vi "Pop Timings Header.vi"(8 "error in (no error)":errorcluster, 11 "Header in":refnum<class "Simulated_Header.lvclass">) -> (0 "error out":errorcluster, 2 "timings header":string, 3 "Header out":refnum<class "Simulated_Header.lvclass">)   [LabVIEW 2018, in "Simulated_Header.lvclass"]
uses:
  Simulated_Header.lvclass
  Simulated_Header.lvclass/Simulated_Header.ctl
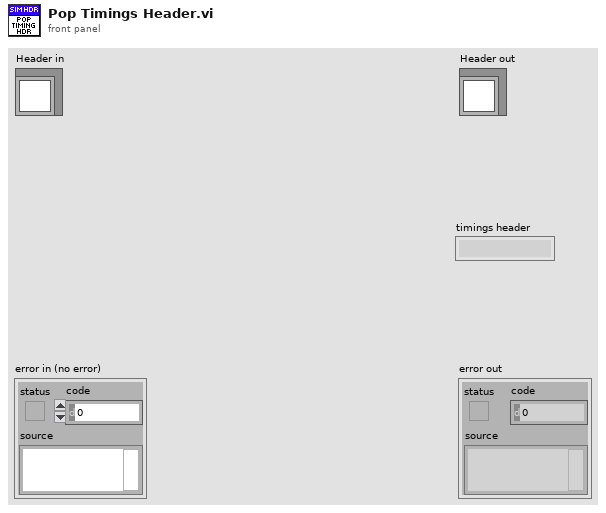
[diagram p1: front panel]
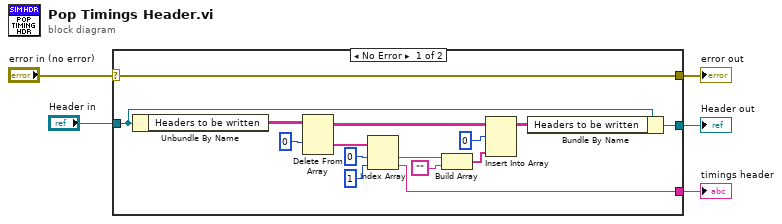
[diagram p0: block diagram]
diagram:
  n1 = case shown="No Error" "error in (no error)" {
    selector: "error in (no error)" -> [w10 w22]
    tunnel: [w10 w22] -> w2
    tunnel: [w9 w21] -> w3
    tunnel: "Header in" -> [w18 w21]
    tunnel: [w8 _] -> w1
    frame No Error {
      n2 = Unbundle By Name(w18) -> ("Headers to be written"=w20:string[][])
      n3 = Delete From Array(array=w20, index (row)=0) -> (deleted portion=w14:string[], array with subset deleted=w17:string[][])  [unwired: 2 in]
      n4 = Index Array(array=w14, index #1=0 ("index (row)"), index #2=1 ("index (row)")) -> (element #1=w6:string, element #2=w8:string)
      n5 = Build Array(w6, "") -> (w11:string[])
      n6 = Insert Into Array(array=w17, index (row)=0, new element=w11) -> (w16:string[][])  [unwired: 1 in]
      n7 = Bundle By Name(cluster=w18, "Headers to be written"=w16) -> (w9:refnum<class "Simulated_Header.lvclass">)
    }
    frame Error {
    }
  }
  "error out" <- w2
  "Header out" <- w3
  "timings header" <- w1
